vi "Remove Object Entry At.vi"(8 "error in":errorcluster, 10 "Index":i32, 11 "Obj Dict in":refnum<class "Object Dictionary.lvclass">) -> (0 "error out":errorcluster, 3 "Obj Dict out":refnum<class "Object Dictionary.lvclass">)   [LabVIEW 2020, in "CANopen.lvlib" / "Object Dictionary.lvclass"]
doc: "Removes the entry at the specified index from the object dictionary."
uses:
  Object Dictionary.lvclass
  Object Dictionary.lvclass/Object Dictionary.ctl
  Ordered-Dictionary/Ordered Object Dictionary/Source/Ordered Object Dictionary.lvclass
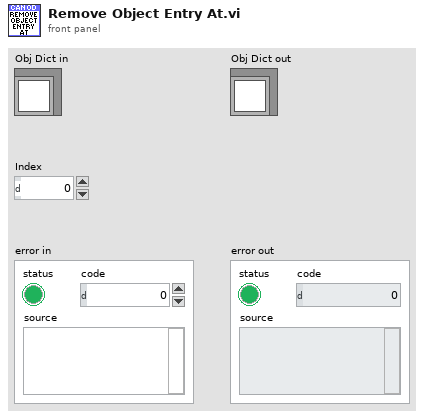
[diagram p1: front panel]
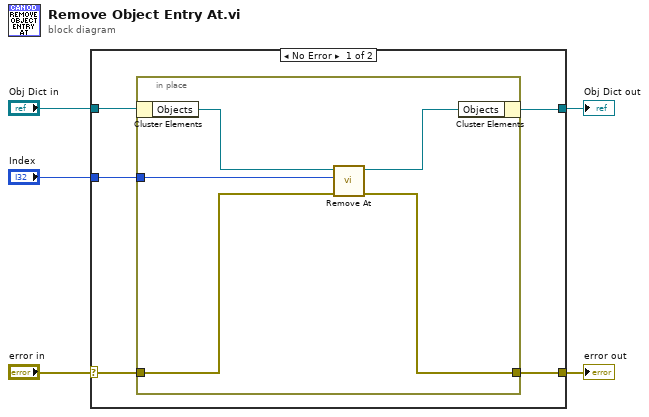
[diagram p0: block diagram]
diagram:
  n1 = case shown="No Error" "error in" {
    selector: "error in" -> [w9 w17]
    tunnel: [w8 w17] -> w2
    tunnel: [w6 w16] -> w4
    tunnel: "Obj Dict in" -> [w7 w16]
    tunnel: "Index" -> [w10 _]
    frame No Error {
      n2 = in-place {
        in-place-border: w10 -> [w15]
        in-place-border: w9 -> [w14]
        in-place-border: [w13] -> w8
        n3 = in-place-cluster #1(w7) -> ("Objects"=w12:refnum<class "Ordered Object Dictionary.lvclass">)
        n4 = call-dynamic "Remove At.vi"("error in"=w14, "Index"=w15, "Ordered Objects Dictionary in"=w12) -> ("error out"=w13:errorcluster, "Ordered Object Dictionary out"=w11:refnum<class "Ordered Object Dictionary.lvclass">)  [unwired: 7 in]
        n5 = in-place-cluster #1("Objects"=w11) -> (w6:refnum<class "Object Dictionary.lvclass">)
      }
    }
    frame Error {
    }
  }
  "Obj Dict out" <- w4
  "error out" <- w2
